vi "Change a folder of vis to have all terminals to Required.vi"() -> ()   [LabVIEW 2013]
panel:
  out "name":string
  out "Array":errorcluster[](array[cluster])
  out "All Files in Dir":path[](array[path])
  in  "Folder Path":path
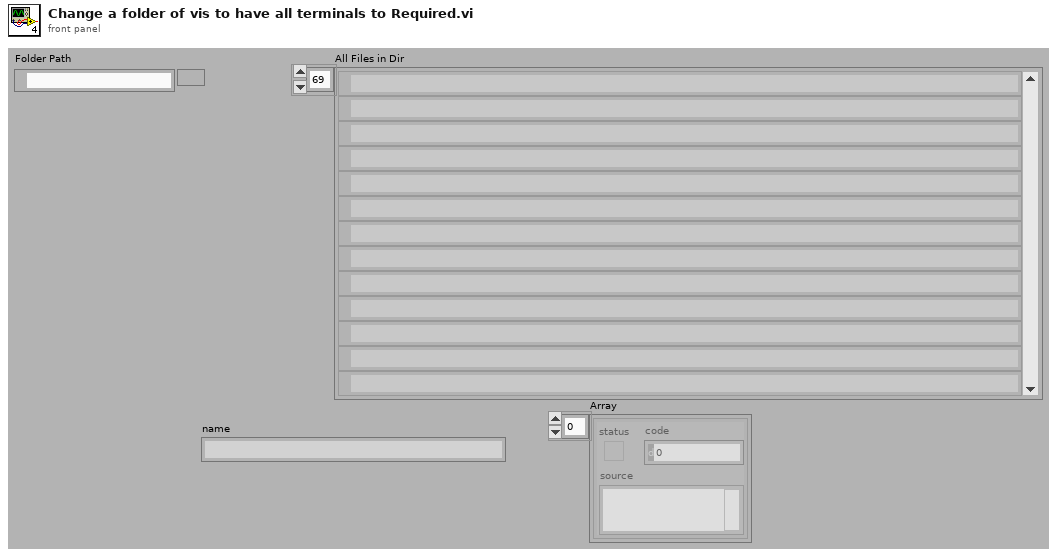
[diagram p1: front panel]
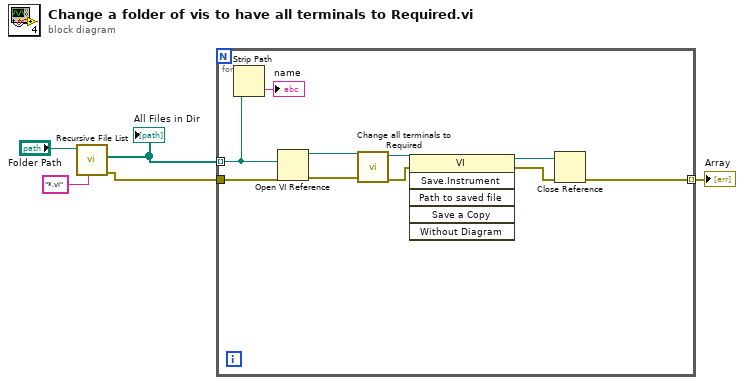
[diagram p0: block diagram]
diagram:
  n1 = call <vilib>:"Recursive File List.vi"("pattern"="*.vi", "Folder Path"="Folder Path") -> ("error out"=w2:errorcluster, "All Files in Dir"=w3:path[])  [unwired: 2 in, 6 out]
  "All Files in Dir" <- w3
  n2 = for {
    tunnel: w3 -> [w7] mode=indexing
    tunnel: w2 -> [w9]
    tunnel: [w8] -> w1 mode=indexing
    n3 = Strip Path(path=w7) -> (name=→"name":string)  [unwired: 1 out]
    n4 = Open VI Reference(vi path=w7, error in (no error)=w9) -> (vi reference=w15:refnum<vi>, error out=w14:errorcluster)  [unwired: 4 out]
    n5 = call "Change all terminals to Required.vi"("error in"=w14, "VI ref to change"=w15) -> ("error out"=w12:errorcluster, "VI ref (dup)"=w13:refnum<vi>)  [unwired: 8 out]
    n6 = invoke class="VI" method="Save.Instrument"(reference=w13, error in=w12) -> (reference out=w11:refnum<vi>, error out=w10:errorcluster)  [unwired: 4 in, 4 out]
    n7 = Close Reference(reference=w11, error in (no error)=w10) -> (error out=w8:errorcluster)
  }
  "Array" <- w1
